vi "get channels.vi"(11 "module configuration in":refnum<class "tag bus configurable plugin module configuration.lvclass">) -> (2 "channels":refnum<class "TBM channel.lvclass">[](array[class]), 3 "module configuration out":refnum<class "tag bus configurable plugin module configuration.lvclass">)   [LabVIEW 2014, in "tag bus configurable plugin module configuration.lvclass"]
doc: "Returns an array of all Channels currently added to this configuration object."
uses:
  tag bus configurable plugin module configuration.lvclass
  <vilib>/NI/Tag Bus Module Framework/channel/TBM channel.lvclass
  tag bus configurable plugin module configuration.lvclass/tag bus configurable plugin module configuration.ctl
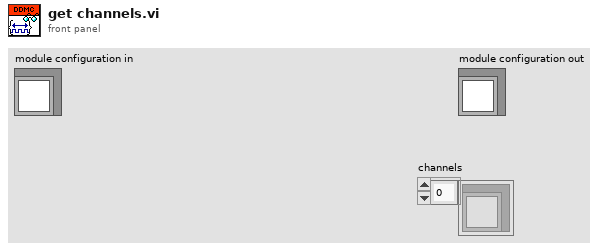
[diagram p1: front panel]
types:
  T1 = typedef "tag bus configurable plugin module configuration.lvclass/Line.ctl" = cluster{"channel":refnum<class "TBM channel.lvclass">}
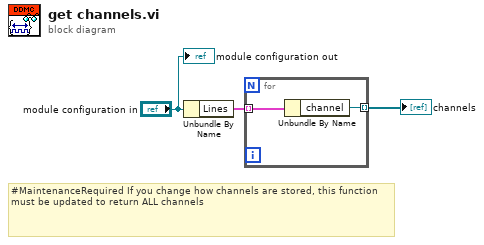
[diagram p0: block diagram]
diagram:
  # "#MaintenanceRequired If you change how channels are stored, this function must be updated to return ALL channels"
  n1 = Unbundle By Name("module configuration in") -> ("Lines"=w2:T1[])
  n2 = for {
    tunnel: w2 -> [w5] mode=indexing
    tunnel: [w4] -> w1 mode=indexing
    n3 = Unbundle By Name(w5) -> ("channel"=w4:refnum<class "TBM channel.lvclass">)
  }
  "channels" <- w1
  "module configuration out" <- "module configuration in"
